vi "PH_uOPA_DelayController.PC Write PSDB.vi"(0 "i ref in":refnum<vi>, 5 "error IO":errorcluster) -> (14 "i ref out":refnum<vi>, 19 "error out":errorcluster)   [LabVIEW 2014, in "PH_uOPA_DelayController.lvlib"]
doc: "This is the proc case which writes data to the PHELIX shot data base."
uses:
  PH_uOPA_DelayController.lvlib
  PH_Basics/PH_StatusHandler/PH_StatusHandler.lvlib
  PH_Devices/PH_TKTDS-30xx/PH_TKTDS-30xx.lvlib
  PH_Basics/PH_PSDBWriter/PH_PSDBWriter.lvlib
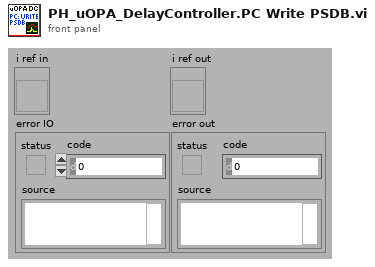
[diagram p1: front panel]
types:
  T1 = typedef "PH_TKTDS-30xx.lvlib/PH_TKTDS-30xx.i attribute.ctl" = cluster{"Default VISA Resource":string, "VISA Resource Name":refnum<visa-resource-name>, "Revision":cluster{"Instrument Driver":string, "Instrument Firmware":string}, "Selftest":cluster{"Result":u32, "Message":string}, "Channels":T2[], "Trigger Configuration":T4, "Acquisition Configuration":T5, "Fetched Waveforms":T6[], "GUI Refs":T7, "State":T8, "Error Message":string, "Allow Prdc Loop?":bool}
  T2 = typedef "PH_TKTDS-30xx.lvlib/PH_TKTDS-30xx.Channel Config.ctl" = cluster{"Channel Name":string, "Input Impedance":string, "Max Input Frequency":string, "Vertical Coupling":i32, "Channel Enabled":bool, "Probe Attenuation":dbl, "Vertical Range":dbl, "Vertical Offset":dbl, "Waveform Limits":T3}
  T3 = typedef "PH_TKTDS-30xx.lvlib/PH_TKTDS-30xx.Waveform Limits.ctl" = cluster{"Start":i32, "End":i32}
  T4 = typedef "PH_TKTDS-30xx.lvlib/PH_TKTDS-30xx.Trigger Config.ctl" = cluster{"Source":string, "Slope":i32, "Level [V]":dbl}
  T5 = typedef "PH_TKTDS-30xx.lvlib/PH_TKTDS-30xx.Acquisition Config.ctl" = cluster{"Time base":dbl, "Record Length":u16, "Start Time":dbl, "Type":i32, "Continuous":bool}
  T6 = typedef "PH_TKTDS-30xx.lvlib/PH_TKTDS-30xx.fetched Waveform.ctl" = cluster{"Source":string, "Actual Points":u32, "Initial X":dbl, "X Increment":dbl, "Waveform Array":dbl[]}
  T7 = typedef "PH_TKTDS-30xx.lvlib/PH_TKTDS-30xx.GUI Refs.ctl" = cluster{"Trigger":refnum<vi>, "Acquisition":refnum<vi>, "State":refnum<vi>, "Delete":refnum<vi>, "Channel to be positioned":refnum<vi>, "Postion":refnum<vi>, "Display Intensity":refnum<vi>, "VISA Resource":refnum<vi>, "Channels":refnum<vi>[], "Graphs":refnum<vi>[]}
  T8 = typedef "PH_StatusHandler.lvlib/PH_StatusHandler.Status.ctl" = i16
  T9 = typedef "PH_PSDBWriter.lvlib/PH_PSDBWriter.String dataset.ctl" = cluster{"name":string, "data":string, "unit":string}
  T10 = typedef "PH_uOPA_DelayController.lvlib/PH_uOPA_DelayController.i attribute.ctl" = cluster{"GUI Refs":cluster{"Current Pump Peak":refnum<vi>, "Current uOPA Peak":refnum<vi>, "Pump Peak":refnum<vi>, "uOPA Peak":refnum<vi>, "uOPA Target":refnum<vi>, "uOPA Limits [%]":refnum<vi>, "sample length":refnum<vi>, "Pump Target":refnum<vi>, "Pump Limit":refnum<vi>, "Pump running":refnum<vi>, "Feedback Control":refnum<vi>, "Control Status":refnum<vi>, "uOPA Mean":refnum<vi>, "Current uOPA Mean":refnum<vi>}, "uOPA Target":dbl, "uOPA Limits [%]":T11, "Sample Length":i32, "Initialize Mean":bool, "Pump Target":dbl, "Pump Limit [%]":dbl, "Feedback Control":bool, "Control Status":T12, "last Mean":dbl, "last direction":T13, "Axis Settings":T14, "Width while feedback":dbl}
  T11 = typedef "PH_uOPA_DelayController.lvlib/PH_uOPA_DelayController.Limit.ctl" = cluster{"low":dbl, "activate":dbl, "fine":dbl}
  T12 = typedef "PH_uOPA_DelayController.lvlib/PH_uOPA_DelayController.Control Status.ctl" = enum32{"off", "Pump off", "calculating", "too low", "activated", "fine"}
  T13 = typedef "PH_Stepmotor_BaseClass.lvlib/PH_Stepmotor_BaseClass.Axis Direction.ctl" = enum16{"forward", "backward"}
  T14 = typedef "PH_Stepmotor_BaseClass.lvlib/PH_Stepmotor_BaseClass.Axis Settings.ctl" = cluster{"Sign change":bool, "Width":dbl, "Calibration":dbl, "Unit":string, "Motor Type":T15, "Unit Width":string, "Unit CF":string}
  T15 = typedef "PH_Stepmotor_BaseClass.lvlib/PH_Stepmotor_BaseClass.Motor Type.ctl" = enum16{"Unspecific", "OWIS 49.120.2633", "OWIS 49.060.1033", "OWIS 43.040.2558", "Diamond Motion 2200 series", "OWIS 49.120.266B.MV6", "Calorimeter", "Linear Stage 1", "MICOS VT-80", "MICOS VT-80 S", "Standa Rotstage nt0.95A", "PUF RA 320.200", "PUF RA 800.200", "PUF RA 800.400", "PUF RA 400.50", "1324.nn.800.50", "1324.n9c.800.50", "1324.nn.320.200", "1324.nn.400.200", "1324.nn.800.200", "1324.nn.400.50", "1324.8c9c.800.50", "1324.8c9c.400.200"}
  T16 = typedef "PH_PSDBWriter.lvlib/PH_PSDBWriter.Boolean dataset.ctl" = cluster{"name":string, "data":bool, "unit":string}
  T17 = typedef "PH_PSDBWriter.lvlib/PH_PSDBWriter.PSDB Dataset.ctl" = cluster{"Version":i32, "2D data Input":T18[], "Boolean Input":T16[], "Image Input":T20[], "Numeric Input":T22[], "String Input":T9[]}
  T18 = typedef "PH_PSDBWriter.lvlib/PH_PSDBWriter.2D dataset.ctl" = cluster{"name":string, "data":dbl[][], "axis description":T19}
  T19 = typedef "PSDB.lvlib/PSDB_AxisDescription.ctl" = cluster{"x axis label":string, "y axis label":string, "x axis unit":string, "y axis unit":string}
  T20 = typedef "PH_PSDBWriter.lvlib/PH_PSDBWriter.Image dataset.ctl" = cluster{"name":string, "data":T21, "unit":string}
  T21 = typedef "IMAQ Image.ctl" = refnum<image>
  T22 = typedef "PH_PSDBWriter.lvlib/PH_PSDBWriter.Numeric dataset.ctl" = cluster{"name":string, "data":dbl, "unit":string}
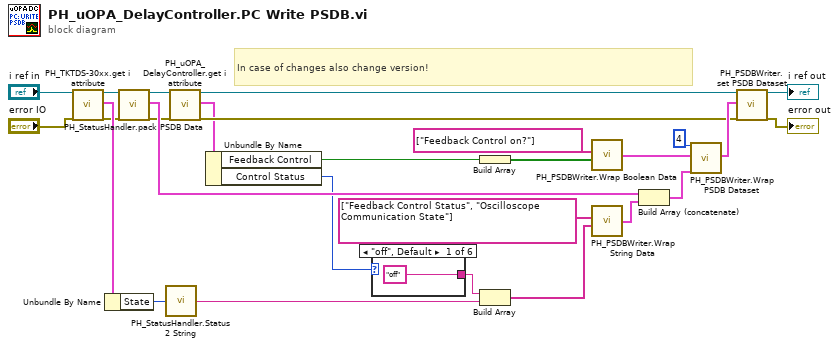
[diagram p0: block diagram]
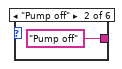
[diagram p2: hidden frame]
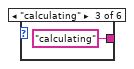
[diagram p3: hidden frame]
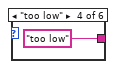
[diagram p4: hidden frame]
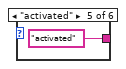
[diagram p5: hidden frame]
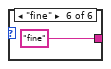
[diagram p6: hidden frame]
diagram:
  # "In case of changes also change version!"
  n1 = call "PH_TKTDS-30xx.get i attribute.vi"("i ref in"="i ref in", "error in (no error)"="error IO") -> ("i ref out"=w26:refnum<vi>, "i attribute"=w27:T1, "error out"=w25:errorcluster)  [unwired: 15 in]
  n2 = Unbundle By Name(w27) -> ("State"=w22:T8)
  n3 = call "PH_StatusHandler.pack PSDB Data.vi"("VI in"=w26, "error in (no error)"=w25) -> ("VI out"=w9:refnum<vi>, "PSDB String Data Array"=w12:T9[], "error out"=w11:errorcluster)  [unwired: 15 in]
  n4 = call "PH_StatusHandler.Status 2 String.vi"("Status"=w22) -> ("Status as string"=w21:string)
  n5 = call "PH_uOPA_DelayController.get i attribute.vi"("i ref in"=w9, "error in (no error)"=w11) -> ("i ref out"=w8:refnum<vi>, "i attribute"=w7:T10, "error out"=w10:errorcluster)  [unwired: 15 in]
  n6 = Unbundle By Name(w7) -> ("Feedback Control"=w5:bool, "Control Status"=w2:T12)
  n7 = case shown="\"off\", Default" w2 {
    tunnel: ["off" "Pump off" "calculating" "too low" "activated" "fine"] -> w1
    frame "off", Default {
    }
    frame "Pump off" {
    }
    frame "calculating" {
    }
    frame "too low" {
    }
    frame "activated" {
    }
    frame "fine" {
    }
  }
  n8 = Build Array(w5) -> (w4:bool[])
  n9 = Build Array(w1, w21) -> (w14:string[])
  n10 = call "PH_PSDBWriter.Wrap Boolean Data.vi"("Data Array"=w4, "Name Array"=string[] ["Feedback Control on?"]) -> ("PSDB Boolean Data Array"=w6:T16[])  [unwired: 2 in]
  n11 = call "PH_PSDBWriter.Wrap String Data.vi"("Data Array"=w14, "Name Array"=string[] ["Feedback Control Status", "Oscilloscope Communication State"]) -> ("PSDB String Data Array"=w16:T9[])  [unwired: 2 in]
  n12 = Build Array (concatenate)(w12, w16) -> (w13:T9[])
  n13 = call "PH_PSDBWriter.Wrap PSDB Dataset.vi"("Version"=4, "Boolean Input"=w6, "String Input"=w13) -> ("PSDB Dataset"=w18:T17)  [unwired: 16 in]
  n14 = call "PH_PSDBWriter.set PSDB Dataset.vi"("VI in"=w8, "PSDB Dataset"=w18, "error in (no error)"=w10) -> ("VI out"=→"i ref out":refnum<vi>, "error out"=→"error out":errorcluster)  [unwired: 15 in]
